vi "Fault_Abnormal_state.vi"() -> ()   [LabVIEW 2016]
panel:
  in  "Abnormal state flag":bool
  in  "Fault state flag":bool
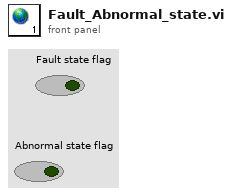
[diagram p1: front panel]
diagram:
